vi "Histogram data rolling array.vi"(8 "error in (no error)":errorcluster, 10 "new data":i32[](array[numeric]), 11 "Rolling array in":T1) -> (0 "error out":errorcluster, 2 "Numofpoints":i32, 3 "Rolling array out":T1)   [LabVIEW 2016]
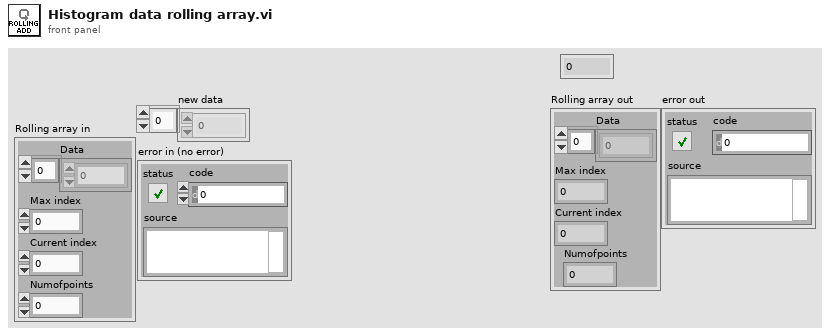
[diagram p1: front panel]
types:
  T1 = cluster{"Data":i32[], "Max index":i32, "Current index":i32, "Numofpoints":i32}
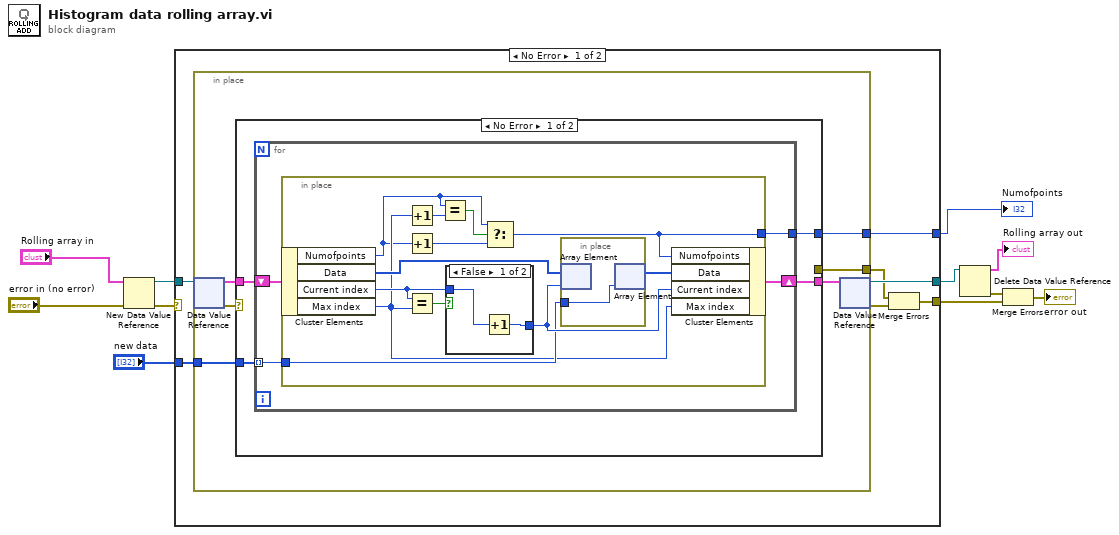
[diagram p0: block diagram]
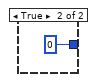
[diagram p2: hidden frame]
diagram:
  n1 = New Data Value Reference(data value="Rolling array in", error in="error in (no error)") -> (data value reference=w10:refnum<data-value>, error out=w5:errorcluster)
  n2 = case shown="No Error" w5 {
    selector: w5 -> [_ w51]
    tunnel: w10 -> [w18 w52]
    tunnel: "new data" -> [w17 _]
    tunnel: [w16 w52] -> w8
    tunnel: [w13 w51] -> w4
    tunnel: [w12 _] -> w1
    frame No Error {
      n3 = in-place {
        in-place-border: [w21] -> w15
        in-place-border: w17 -> [w20]
        in-place-border: [w19] -> w12
        n4 = in-place-dvr #1(w18) -> (w24:T1, w22:errorcluster)
        n5 = case shown="No Error" w22 {
          selector: w22 -> [_ w50]
          tunnel: w24 -> [w28 w49]
          tunnel: [w27 w49] -> w23
          tunnel: [_ w50] -> w21
          tunnel: w20 -> [w26 _]
          tunnel: [w25 _] -> w19
          frame No Error {
            n6 = for {
              tunnel: w26 -> [w30] mode=indexing
              shift-right: [w31] -> w27
              shift-left: w28 -> [w32]
              tunnel: [w29] -> w25
              n7 = in-place {
                in-place-border: w30 -> [w39]
                in-place-border: [w33] -> w29
                n8 = in-place-cluster #2(w32) -> ("Numofpoints"=w34:i32, "Data"=w44:i32[], "Current index"=w43:i32, "Max index"=w38:i32)
                n9 = Increment(x=w38) -> (x+1=w37:i32)
                n10 = Increment(x=w34) -> (x+1=w35:i32)
                n11 = Equal?(x=w43, y=w38) -> (x = y?=w41:bool)
                n12 = Equal?(x=w34, y=w37) -> (x = y?=w36:bool)
                n13 = case shown="False" w41 {
                  tunnel: [w46 0] -> w42
                  tunnel: w43 -> [w45 _]
                  frame False {
                    n14 = Increment(x=w45) -> (x+1=w46:i32)
                  }
                  frame True {
                  }
                }
                n15 = Select(t=w34, s=w36, f=w35) -> (s? t:f=w33:i32)
                n16 = in-place {
                  in-place-border: w39 -> [w48]
                  n17 = in-place-array #3(w44, w42) -> ()  [unwired: 1 out]
                  n18 = in-place-array #3(w48) -> (w40:i32[])  [unwired: 1 out]
                }
                n19 = in-place-cluster #2("Numofpoints"=w33, "Data"=w40, "Current index"=w42, "Max index"=w38) -> (w31:T1)
              }
            }
          }
          frame Error {
          }
        }
        n20 = in-place-dvr #1(w23) -> (w16:refnum<data-value>, w14:errorcluster)
      }
      n21 = Merge Errors(w15, w14) -> (w13:errorcluster)
    }
    frame Error {
    }
  }
  "Numofpoints" <- w1
  n22 = Delete Data Value Reference(data value reference=w8) -> (data value=→"Rolling array out":T1, error out=w3:errorcluster)  [unwired: 1 in]
  n23 = Merge Errors(w3, w4) -> (→"error out":errorcluster)
